vi "Public Key File Authentication.vi"(7 "Keys":cluster{"Private":path, "Public":path}={"Private"=path "", "Public"=path ""}, 8 "Error In":errorcluster, 9 "Passphrase":string, 10 "Username":string, 11 "Session In":refnum<class "Session.lvclass">) -> (0 "Error Out":errorcluster, 3 "Sesssion Out":refnum<class "Session.lvclass">)   [LabVIEW 2021, in "Field_RnD_Services_LIBSSH2_Toolkit.lvlib" / "Session.lvclass"]
doc: "Authenticates this session using a public-private key pair saved in files on the local machine."
uses:
  Session.lvclass
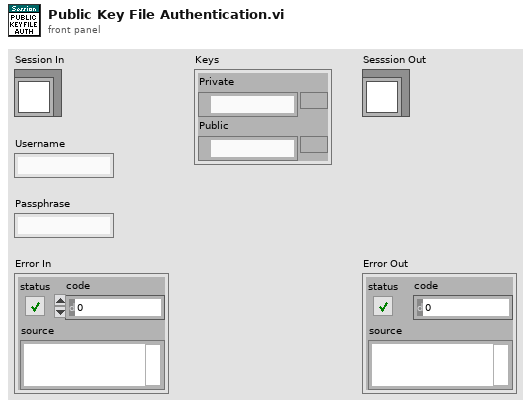
[diagram p1: front panel]
types:
  T1 = enum16{"open", "replace", "create", "open or create", "replace or create", "replace or create with confirmation"}
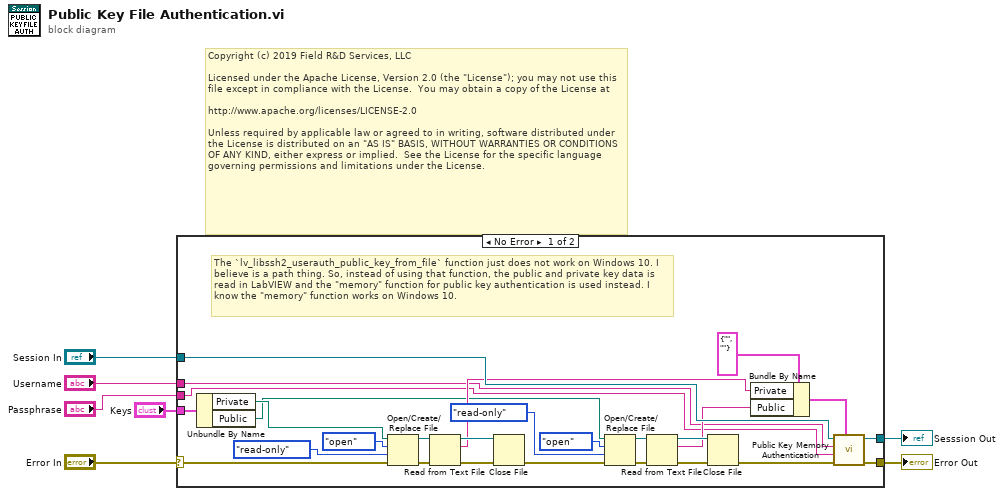
[diagram p0: block diagram]
diagram:
  # "Copyright (c) 2019 Field R&D Services, LLC\n\nLicensed under the Apache License, Version 2.0 (the \"License\"); you may not use this file except in compliance with the License.  You may obtain a copy of the License at\n\nhttp://www.apache.org/licenses/LICENSE-2.0\n\nUnless required by applicable law or agreed to in writing, software distributed under the License is distributed on an \"AS IS\" BASIS, WITHOUT WARRANTIES OR CONDITIONS OF ANY KIND, either express or implied.  See the License for the specific language governing permissions and limitations under the License."
  n1 = case shown="No Error" "Error In" {
    selector: "Error In" -> [w28 w36]
    tunnel: [w23 w36] -> w6
    tunnel: "Session In" -> [w25 w35]
    tunnel: [w24 w35] -> w4
    tunnel: "Username" -> [w8 _]
    tunnel: "Passphrase" -> [w9 _]
    tunnel: "Keys" -> [w30 _]
    frame No Error {
      # "The `lv_libssh2_userauth_public_key_from_file` function just does not work on Windows 10. I believe is a path thing. So, instead of using that function, the public and private key data is read in LabVIEW and the \"memory\" function for public key authentication is used instead. I know the \"memory\" function works on Windows 10."
      n2 = Unbundle By Name(w30) -> ("Private"=w29:path, "Public"=w12:path)
      n3 = Open/Create/Replace File(file path (use dialog)=w29, error in=w28, operation (0:open)=T1."open", access (0:read/write)=enum16{"read/write", "read-only", "write-only"}."read-only") -> (refnum out=w31:refnum<file>, error out=w32:errorcluster)  [unwired: 2 in, 1 out]
      n4 = Read from Text File(file (use dialog)=w31, error in=w32) -> (refnum out=w34:refnum<file>, text=w20:string, error out=w33:errorcluster)  [unwired: 2 in, 1 out]
      n5 = Close File(refnum=w34, error in=w33) -> (error out=w13:errorcluster)  [unwired: 1 out]
      n6 = Open/Create/Replace File(file path (use dialog)=w12, error in=w13, operation (0:open)=T1."open", access (0:read/write)=enum16{"read/write", "read-only", "write-only"}."read-only") -> (refnum out=w16:refnum<file>, error out=w17:errorcluster)  [unwired: 2 in, 1 out]
      n7 = Read from Text File(file (use dialog)=w16, error in=w17) -> (refnum out=w19:refnum<file>, text=w11:string, error out=w18:errorcluster)  [unwired: 2 in, 1 out]
      n8 = Close File(refnum=w19, error in=w18) -> (error out=w10:errorcluster)  [unwired: 1 out]
      n9 = Bundle By Name(cluster=cluster{"Private":string, "Public":string} {"Private"="", "Public"=""} ("Keys"), "Private"=w20, "Public"=w11) -> (w21:cluster{"Private":string, "Public":string})
      n10 = call "Public Key Memory Authentication.vi"("Keys"=w21, "Error In"=w10, "Passphrase"=w9, "Username"=w8, "Session In"=w25) -> ("Error Out"=w23:errorcluster, "Sesssion Out"=w24:refnum<class "Session.lvclass">)  [unwired: 5 in]
    }
    frame Error {
    }
  }
  "Sesssion Out" <- w4
  "Error Out" <- w6
